vi "ConvertToLakeShore340Format.vi"() -> ()   [LabVIEW 2016]
panel:
  out "XY Graph":cluster{dbl[], dbl[]}(graph)
  in  "Row format string":string="%3d%9.5f%14.3f\\n"
  in  "Resistance column":i32=1
  in  "Temperature column":i32
  in  "transpose (no:F)":bool=TRUE
  in  "delimiter (Tab)":string="   "
  in  "Number of header lines":i32=3
  out "text":string="Sensor Model:   CX-1030-SD-0.3L\nSerial Number:  X44163\nData Format:    4      (Log Ohms/Kelvin)\nSetPoint Limit: 325.0      (Kelvin)\nTemperature coefficient:  1 (Negative)\nNumber of Breakpoints:   179\n\nNo.   Units      Temperature (K)\n\n  1  1.64294       325.000\n  2  1.64798       319.000\n  3  1.65270       313.500\n  4  1.65751       308.000\n  5  1.66243       302.500\n  6  1.66745       297.000\n  7  1.67259       291.500\n  8  1.67783       286.000\n  9  1.68319       280.500\n 10  1.68867       275.000\n 11  1.69428       269.500\n 12  1.70001       264.000\n 13  1.70587       258.500\n 14  1.71187       253.000\n 15  1.71801       247.500\n 16  1.72429       242.000\n 17  1.73073       236.500\n 18  1.73732       231.000\n 19  1.74345       226.000\n 20  1.74971       221.000\n 21  1.75612       216.000\n 22  1.76268       211.000\n 23  1.76940       206.000\n 24  1.77627       201.000\n 25  1.78331       196.000\n 26  1.79052       191.000\n 27  1.79792       186.000\n 28  1.80550       181.000\n 29  1.81329       176.000\n 30  1.82127       171.000\n 31  1.82865       166.500\n 32  1.83620       162.000\n 33  1.84395       157.500\n 34  1.85189       153.000\n 35  1.86005       148.500\n 36  1.86842       144.000\n 37  1.87702       139.500\n 38  1.88587       135.000\n 39  1.89498       130.500\n 40  1.90332       126.500\n 41  1.91189       122.500\n 42  1.92070       118.500\n 43  1.92979       114.500\n 44  1.93916       110.500\n 45  1.94883       106.500\n 46  1.95884       102.500\n 47  1.96659        99.500\n 48  1.97319        97.000\n 49  1.97995        94.500\n 50  1.98687        92.000\n 51  1.99396        89.500\n 52  2.00124        87.000\n 53  2.00871        84.500\n 54  2.01639        82.000\n 55  2.02430        79.500\n 56  2.03080        77.500\n 57  2.03744        75.500\n 58  2.04426        73.500\n 59  2.05126        71.500\n 60  2.05845        69.500\n 61  2.06584        67.500\n 62  2.07344        65.500\n 63  2.08126        63.500\n 64  2.08933        61.500\n 65  2.09807        59.400\n 66  2.10581        57.600\n 67  2.11379        55.800\n 68  2.12201        54.000\n 69  2.13051        52.200\n 70  2.13929        50.400\n 71  2.14838        48.600\n 72  2.15781        46.800\n 73  2.16649        45.200\n 74  2.17546        43.600\n 75  2.18475        42.000\n 76  2.19439        40.400\n 77  2.20440        38.800\n 78  2.21482        37.200\n 79  2.22498        35.700\n 80  2.23555        34.200\n 81  2.24657        32.700\n 82  2.25730        31.300\n 83  2.26849        29.900\n 84  2.28019        28.500\n 85  2.29157        27.200\n 86  2.30346        25.900\n 87  2.31595        24.600\n 88  2.32808        23.400\n 89  2.34081        22.200\n 90  2.35312        21.100\n 91  2.36488        20.100\n 92  2.37412        19.350\n 93  2.38241        18.700\n 94  2.39100        18.050\n 95  2.39992        17.400\n 96  2.40848        16.800\n 97  2.41737        16.200\n 98  2.42662        15.600\n 99  2.43627        15.000\n100  2.44551        14.450\n101  2.45514        13.900\n102  2.46521        13.350\n103  2.47479        12.850\n104  2.48480        12.350\n105  2.49530        11.850\n106  2.50632        11.350\n107  2.51677        10.900\n108  2.52772        10.450\n109  2.53927        10.000\n110  2.55146         9.550\n111  2.56438         9.100\n112  2.57656         8.700\n113  2.58944         8.300\n114  2.60314         7.900\n115  2.61773         7.500\n116  2.63137         7.150\n117  2.64586         6.800\n118  2.66136         6.450\n119  2.67800         6.100\n120  2.69435         5.780\n121  2.71193         5.460\n122  2.72973         5.160\n123  2.74894         4.860\n124  2.76984         4.560\n125  2.79112         4.280\n126  2.81265         4.020\n127  2.83062         3.820\n128  2.84787         3.640\n129  2.86634         3.460\n130  2.88508         3.290\n131  2.90401         3.130\n132  2.92435         2.970\n133  2.94633         2.810\n134  2.96862         2.660\n135  2.99273         2.510\n136  3.01724         2.370\n137  3.04389         2.230\n138  3.07100         2.100\n139  3.10062         1.970\n140  3.13074         1.850\n141  3.16384         1.730\n142  3.20061         1.610\n143  3.23821         1.500\n144  3.28018         1.390\n145  3.32315         1.290\n146  3.36149         1.210\n147  3.38762         1.160\n148  3.40968         1.120\n149  3.43301         1.080\n150  3.45776         1.040\n151  3.48407         1.000\n152  3.51212         0.960\n153  3.54211         0.920\n154  3.57019         0.885\n155  3.60007         0.850\n156  3.63206         0.815\n157  3.66638         0.780\n158  3.70336         0.745\n159  3.73751         0.715\n160  3.77404         0.685\n161  3.81340         0.655\n162  3.85594         0.625\n163  3.90212         0.595\n164  3.95249         0.565\n165  4.00785         0.535\n166  4.05856         0.510\n167  4.10245         0.490\n168  4.14486         0.472\n169  4.19034         0.454\n170  4.23384         0.438\n171  4.28035         0.422\n172  4.33035         0.406\n173  4.38405         0.390\n174  4.44177         0.374\n175  4.50377         0.358\n176  4.57044         0.342\n177  4.64226         0.326\n178  4.71045         0.312\n179  4.77490         0.300\n"
  in  "Header Format String":string="Sensor Model:   CX-1030-SD-0.3L\nSerial Number:  X07887\nData Format:    4      (Log Ohms/Kelvin)\nSetPoint Limit: 325.0      (Kelvin)\nTemperature coefficient:  1 (Negative)\nNumber of Breakpoints:   %d\n\nNo.   Units      Temperature (K)\n\n"
  in  "Output Path":path=path "D:/LabviewLib/beta/magnet lab/Sensors/X07887.340"
  in  "Input file":path=path "E:/thermometers/probes/X07887.dat"
  # "Input"
  # "Output"
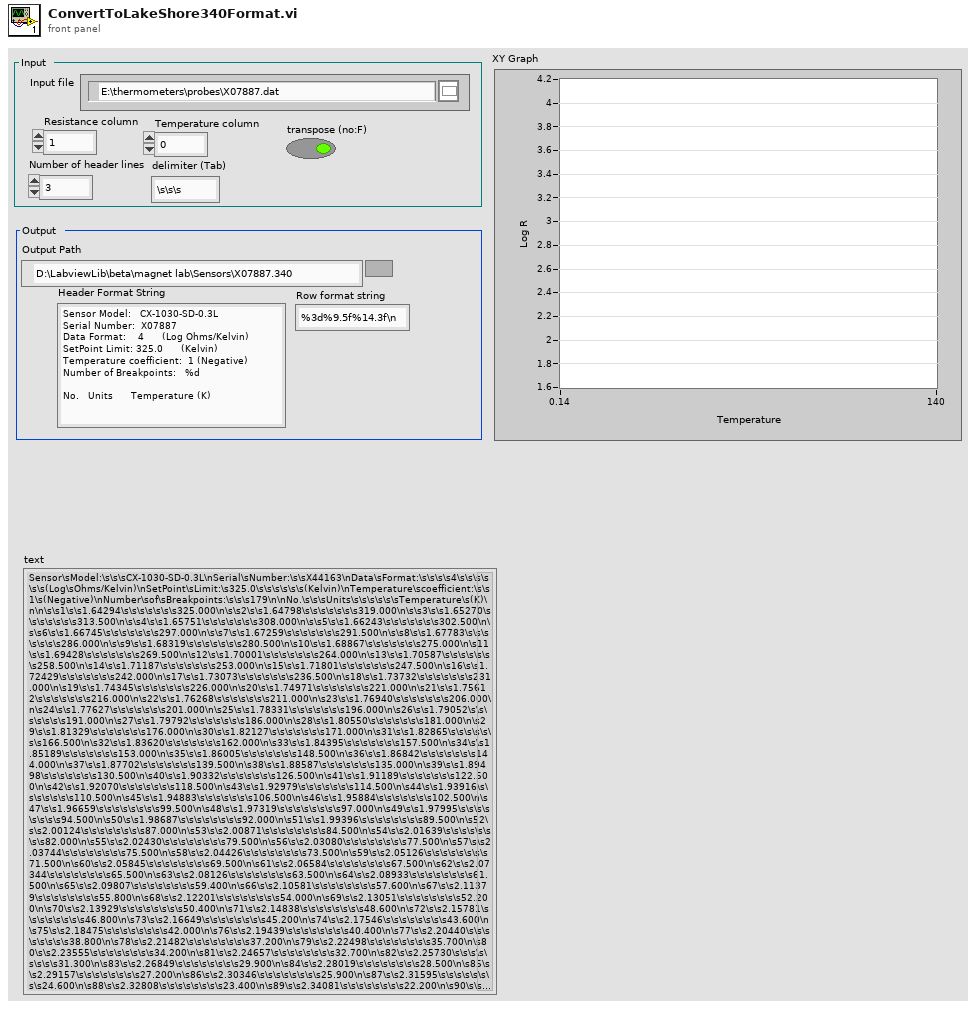
[diagram p1: front panel]
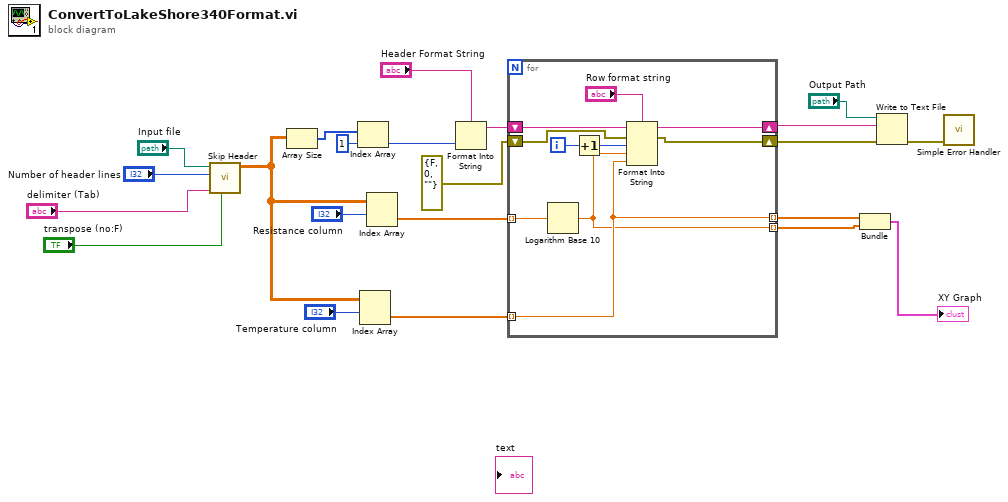
[diagram p0: block diagram]
diagram:
  n1 = call "Skip Header.vi"("transpose (yes:T)"="transpose (no:F)", "delimiter (Tab)"="delimiter (Tab)", "number of header lines"="Number of header lines", "Input File Name"="Input file") -> ("all rows"=w13:dbl[][])  [unwired: 1 in, 6 out]
  n2 = Array Size(array=w13) -> (size(s)=w18:i32[])
  n3 = Index Array(array=w18, index=1) -> (element=w4:i32)
  n4 = Index Array(array=w13, index (row)="Temperature column") -> (element=w12:dbl[])  [unwired: 1 in]
  n5 = Index Array(array=w13, index (row)="Resistance column") -> (element=w11:dbl[])  [unwired: 1 in]
  n6 = Format Into String(format string="Header Format String", w4) -> (resulting string=w10:string)  [unwired: 2 in, 1 out]
  n7 = for {
    tunnel: w12 -> [w24] mode=indexing
    tunnel: w11 -> [w29] mode=indexing
    shift-right: [w27] -> w9
    shift-left: w10 -> [w30]
    shift-right: [w25] -> w7
    shift-left: errorcluster {"status"=FALSE, "code"=0, "source"=""} ("error IO") -> [w26]
    tunnel: [w24] -> w3 mode=indexing
    tunnel: [w23] -> w2 mode=indexing
    i -> [w32]
    n8 = Logarithm Base 10(1:w29) -> (0:w23:dbl)
    n9 = Increment(x=w32) -> (x+1=w31:i32)
    n10 = Format Into String(format string="Row format string", initial string=w30, error in=w26, w31, w23, w24) -> (resulting string=w27:string, error out=w25:errorcluster)
  }
  n11 = Bundle(w3, w2) -> (→"XY Graph":cluster{dbl[], dbl[]})  [unwired: 1 in]
  n12 = Write to Text File(file (use dialog)="Output Path", text=w9, error in=w7) -> (error out=w6:errorcluster)  [unwired: 3 out]
  n13 = call <vilib>:"Simple Error Handler.vi"("error in (no error)"=w6) -> ()  [unwired: 1 in, 8 out]
